vi "Trajectory Test.vi"() -> ()   [LabVIEW 2018]
uses:
  Controls/Robot State.ctl
  Controls/Robot Pivot Motion Commands.ctl
  Controls/Pivot Motor Commands.ctl
  Controls/Robot Drive Mode.ctl
  Controls/Climb Motor Commands.ctl
  Controls/Arm Motor Commands.ctl
  Controls/Ball Motor Commands.ctl
  Controls/Dics Eject Command.ctl
  Controls/Lift Motor Commands.ctl
  Controls/Grip Motor Commands.ctl
  Controls/Enable Actions.ctl
  Global Variables/Trajectory Enabled.vi
  Global Variables/Robot State.vi
panel:
  in  "Trajectory Enabled":bool
  out "Robot State":T1
  in  "stop":bool
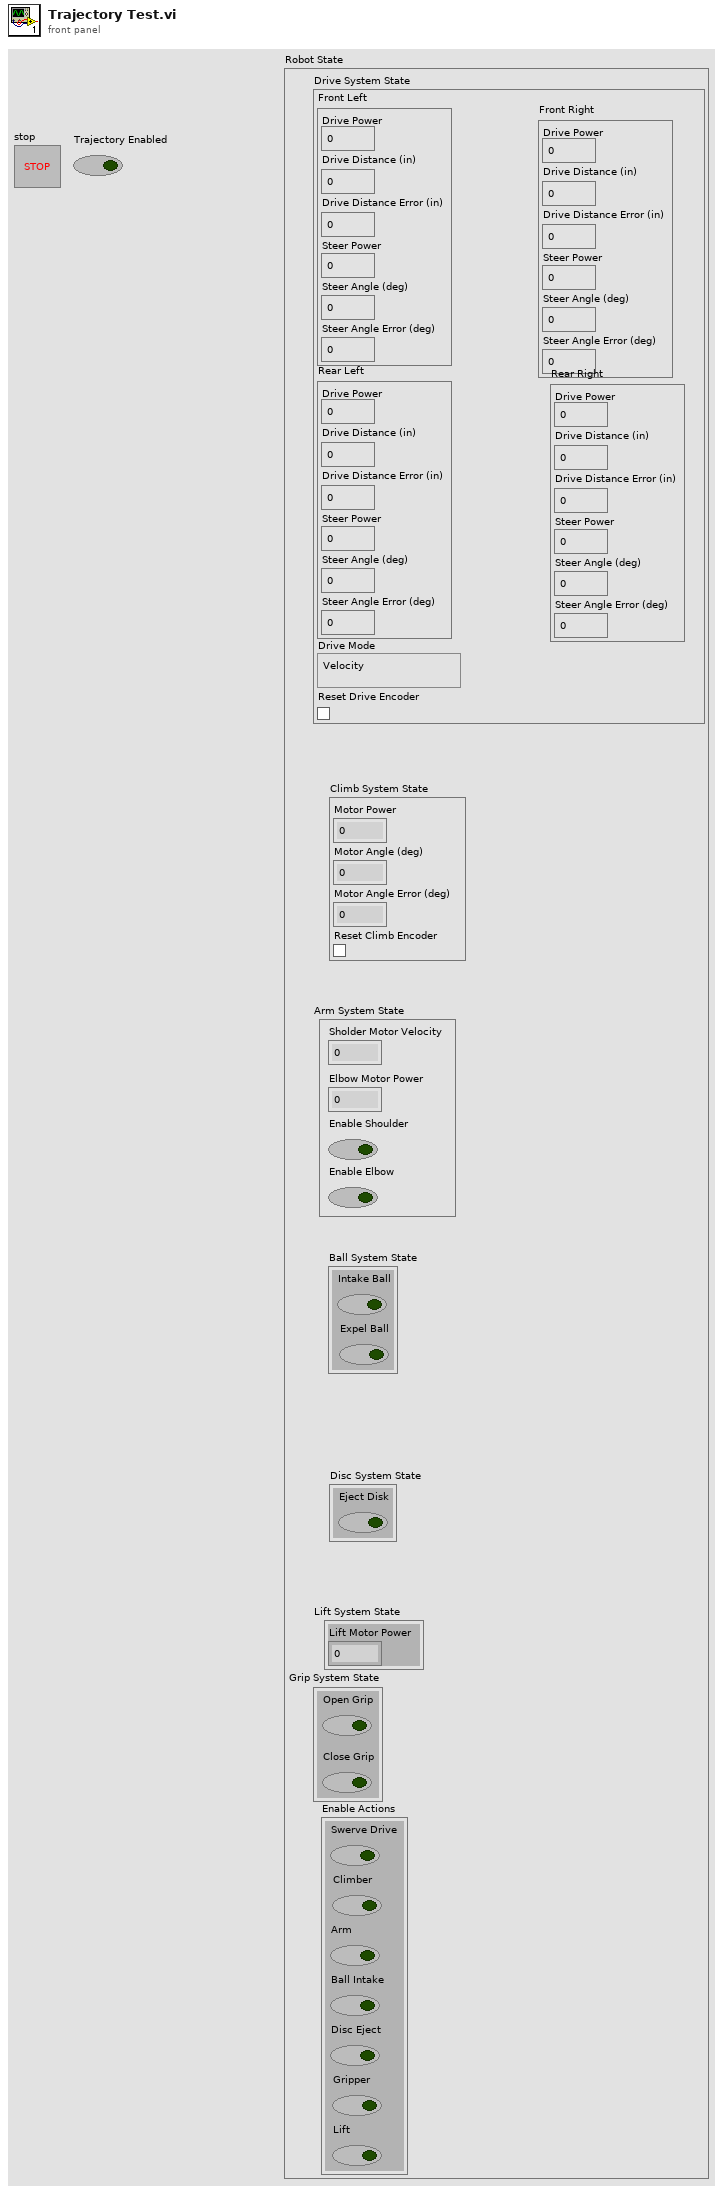
[diagram p1: front panel]
types:
  T1 = typedef "Robot State.ctl" = cluster{"Drive System State":T2, "Climb System State":T5, "Arm System State":T6, "Ball System State":T7, "Disc System State":T8, "Lift System State":T9, "Grip System State":T10, "Enable Actions":T11}
  T2 = typedef "Robot Pivot Motion Commands.ctl" = cluster{"Front Right":T3, "Front Left":T3, "Rear Left":T3, "Rear Right":T3, "Drive Mode":T4, "Reset Drive Encoder":bool}
  T3 = typedef "Pivot Motor Commands.ctl" = cluster{"Drive Power":dbl, "Drive Distance (in)":dbl, "Drive Distance Error (in)":dbl, "Steer Power":dbl, "Steer Angle (deg)":dbl, "Steer Angle Error (deg)":dbl}
  T4 = typedef "Robot Drive Mode.ctl" = enum16{"Velocity", "Distance"}
  T5 = typedef "Climb Motor Commands.ctl" = cluster{"Motor Power":dbl, "Motor Angle (deg)":dbl, "Motor Angle Error (deg)":dbl, "Reset Climb Encoder":bool}
  T6 = typedef "Arm Motor Commands.ctl" = cluster{"Enable Shoulder":bool, "Enable Elbow":bool, "Elbow Motor Power":dbl, "Sholder Motor Velocity":dbl}
  T7 = typedef "Ball Motor Commands.ctl" = cluster{"Intake Ball":bool, "Expel Ball":bool}
  T8 = typedef "Dics Eject Command.ctl" = cluster{"Eject Disk":bool}
  T9 = typedef "Lift Motor Commands.ctl" = cluster{"Lift Motor Power":dbl}
  T10 = typedef "Grip Motor Commands.ctl" = cluster{"Open Grip":bool, "Close Grip":bool}
  T11 = typedef "Enable Actions.ctl" = cluster{"Swerve Drive":bool, "Climber":bool, "Arm":bool, "Ball Intake":bool, "Disc Eject":bool, "Gripper":bool, "Lift":bool}
  T12 = typedef "Robot Actions.ctl" = cluster{"Durations":dbl, "Robot State":T1}
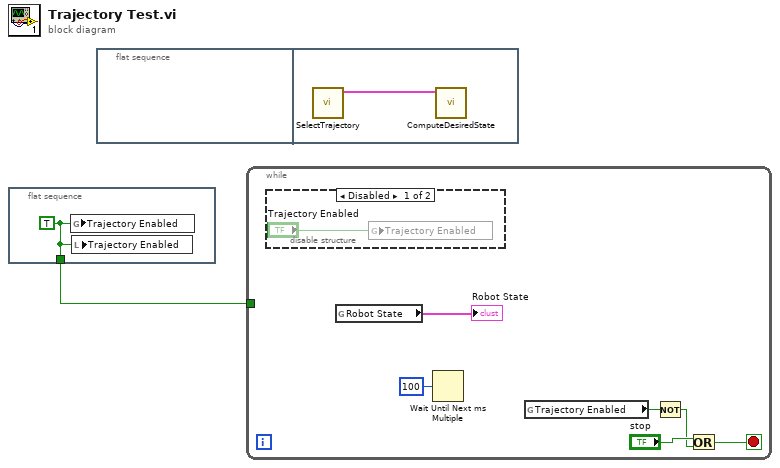
[diagram p0: block diagram]
diagram:
  n1 = flat-sequence {
    tunnel: [w2] -> w1
    frame #0 {
      w2 = TRUE ("Trajectory Enabled")
      n2 = global write "Trajectory Enabled.vi" "Trajectory Enabled"(w2) -> ()
      n3 = local write "Trajectory Enabled"(w2) -> ()
    }
  }
  n4 = flat-sequence {
    frame #0 {
    }
    frame #1 {
      n5 = call "SelectTrajectory.vi"() -> ("Robot Action Array"=w3:T12[])  [unwired: 11 in]
      n6 = call "ComputeDesiredState.vi"("Robot Action Array"=w3) -> ()  [unwired: 11 in]
    }
  }
  n7 = while {
    tunnel: w1 -> [_]
    stop <- w5 stop-if-true
    n8 = disable-structure shown="Disabled" {
      frame Disabled {
        n9 = global write "Trajectory Enabled.vi" "Trajectory Enabled"("Trajectory Enabled") -> ()
      }
      frame Enabled {
      }
    }
    n10 = global read "Robot State.vi" "Robot State"() -> (→"Robot State":T1)
    n11 = Wait Until Next ms Multiple(millisecond multiple=u32 100) -> ()  [unwired: 1 out]
    n12 = global read "Trajectory Enabled.vi" "Trajectory Enabled"() -> (w6:bool)
    n13 = Not(x=w6) -> (.not. x?=w4:bool)
    n14 = Or(x="stop", y=w4) -> (x .or. y?=w5:bool)
  }
